vi "PXImc Custom Device.Async.vi"(10 "Parameters":variant, 11 "Process":refnum<class "Process.lvclass">) -> ()   [LabVIEW 2016, in "PXImc Custom Device Engine.lvlib"]
uses:
  PXImc Custom Device Engine.lvlib
  <vilib>/NI/NIVS Inline Async API/_VS Inline Async API/Process/Process.lvclass
  Shared/Compiled.Settings.ctl
  PXImc Router/Controls/Target Type.ctl
  PXImc Router/Controls/Router - Configuration.ctl
  PXImc Router/Controls/Router/Node Block R-W Properties.ctl
  PXImc Router/Controls/Router/Block Properties.ctl
  PXImc Router/Controls/Router/Router - PXImc Properties.ctl
  PXImc Router/Controls/Router/Router - PXImc Card Properties.ctl
  PXImc Router/Controls/Node Data.ctl
  PXImc Router/Controls/Node/Node - PXImc Parameters.ctl
  PXImc Router/Controls/Node/Node - Writer Data.ctl
  PXImc Router/Controls/Node/Node Ch Properties.ctl
  PXImc Router/Controls/Data Type.ctl
  PXImc Router/Controls/Node/Node - Readers Data.ctl
  PXImc Router/Controls/Node/Node - Reader Data.ctl
  <vilib>/NI/NIVS Inline Async API/_VS Inline Async API/Process/Process.lvclass/Process.ctl
  <vilib>/NI/NIVS Inline Async API/_Data Access Engine/Access Type Classes/Read/Read.lvclass/Read.ctl
  <vilib>/NI/NIVS Inline Async API/_Data Access Engine/Access Type Classes/Write/Write.lvclass/Write.ctl
  <vilib>/NI/NIVS Inline Async API/_Data Access Engine/Data Access Engine/Methods/Write.Data.vi
  <vilib>/NI/NIVS Inline Async API/_Data Access Engine/Data Access Engine/Methods/Read.Data.vi
  <vilib>/NI/NIVS Inline Async API/_VS Inline Async API/Process/Data Member Access/Read Data Access.vi
  <vilib>/NI/NIVS Inline Async API/_VS Inline Async API/Error Handling Process/SubVIs/Error.ConvertArray.vi
  <vilib>/NI/NIVS Inline Async API/_Data Access Engine/Access Type Classes/Write/Write.ProcessData.vi
  <vilib>/NI/NIVS Inline Async API/_Data Access Engine/Access Type Classes/Read/Read.ProcessData.vi
  <vilib>/NI/NIVS Inline Async API/_Data Access Engine/Data Access Engine/Methods/Read.Lookup.vi
  <vilib>/NI/NIVS Inline Async API/_Data Access Engine/Data Access Engine/Methods/Write.Lookup.vi
  Shared/Constants.vi
  <vilib>/NI/NIVS Inline Async API/_Data Access Engine/Data Access Engine/Data Access Engine.lvclass
  PXImc Router/PXImc Router.lvlib
  Shared/PXImc Custom Device Shared.lvlib
  <vilib>/nisyscfg/nisyscfg.lvlib
  <resource>/objmgr/nicriosae.rc
  <resource>/objmgr/nisysapi.rc
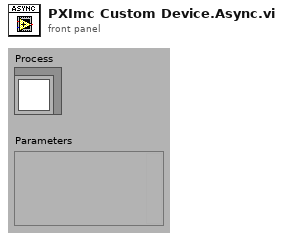
[diagram p1: front panel]
types:
  T1 = enum16{"Create File", "Log Message", "Log Error", "Log TimeStamp", "Close File"}
  T2 = typedef "PXImc Custom Device Shared.lvlib/Compiled.Settings.ctl" = cluster{"Target Type":T3, "Router Properties":T4, "Node Data":T9, "Configuration Folder Path":path}
  T3 = typedef "PXImc Router.lvlib/Target Type.ctl" = enum16{"Router", "Node"}
  T4 = typedef "PXImc Router.lvlib/Router - Configuration.ctl" = cluster{"Target Type":T3, "Master Table Ref":refnum<data-value>, "Master Table Size (Bytes)":u32, "Node Properties":T5[], "Router - PXImc Properties":T7}
  T5 = typedef "PXImc Router.lvlib/Node Block R-W Properties.ctl" = cluster{"Node ID":u32, "# Reading Blocks":u32, "Node Writing Block":T6, "Node Reading Blocks":T6[]}
  T6 = typedef "PXImc Router.lvlib/Block Properties.ctl" = cluster{"Offset":u32, "Size (Bytes)":u32}
  T7 = typedef "PXImc Router.lvlib/Router - PXImc Properties.ctl" = cluster{"PXImc Cards Properties":T8[], "Connection Timeout (s)":dbl, "Readers Buffer Size":u64}
  T8 = typedef "PXImc Router.lvlib/Router - PXImc Card Properties.ctl" = cluster{"PXImc Resource Name":string, "Reader - PXImc Session Ref":refnum<k21>, "Writer - PXImc Session Ref":refnum<k21>, "Reader Conn ID":u16, "Writer Conn ID":u16}
  T9 = typedef "PXImc Router.lvlib/Node Data.ctl" = cluster{"Node Name":string, "PXImc Parameters":T10, "Local Data":T11, "Imported Data":T14}
  T10 = typedef "PXImc Router.lvlib/Node - PXImc Parameters.ctl" = cluster{"Resource Name":string, "Connection Timeout (s)":dbl, "Readers Buffer Size":u64, "Node PXImc Reader Conn Id":u16, "Node PXImc Writer Conn Id":u16, "Writer PXImc Session":refnum<k21>, "Reader PXImc Session":refnum<k21>}
  T11 = typedef "PXImc Router.lvlib/Node - Writer Data.ctl" = cluster{"Flattened Byte Buffer Ref":string, "Noder ID":u32, "Master Table Offest":u32, "Byte Buffer Size":u32, "Node Local Channels":T12[], "Node Local Channels Table":string[][]}
  T12 = typedef "PXImc Router.lvlib/Node Ch Properties.ctl" = cluster{"Name":string, "Value":dbl, "Data Type":T13}
  T13 = typedef "PXImc Router.lvlib/Data Type.ctl" = enum16{"Boolean", "SGL", "DBL", "I8", "I16", "I32", "I64", "U8", "U16", "U32", "U64"}
  T14 = typedef "PXImc Router.lvlib/Node - Readers Data.ctl" = cluster{"Flattened Byte Buffer Ref":string, "Byte Buffer Size":u64, "Readers Data Array":T15[], "Node Imported Channels Table":string[][]}
  T15 = typedef "PXImc Router.lvlib/Node - Reader Data.ctl" = cluster{"Noder ID":u32, "Master Table Offest":u32, "Byte Buffer Size":u64, "Node Imported Channels":T12[]}
  T16 = typedef "Data Access Engine.lvlib/Data Access Engine.lvclass/Write.DVR.ctl" = refnum<data-value>
  T17 = typedef "Data Access Engine.lvlib/Data Access Engine.lvclass/Read.DVR.ctl" = refnum<data-value>
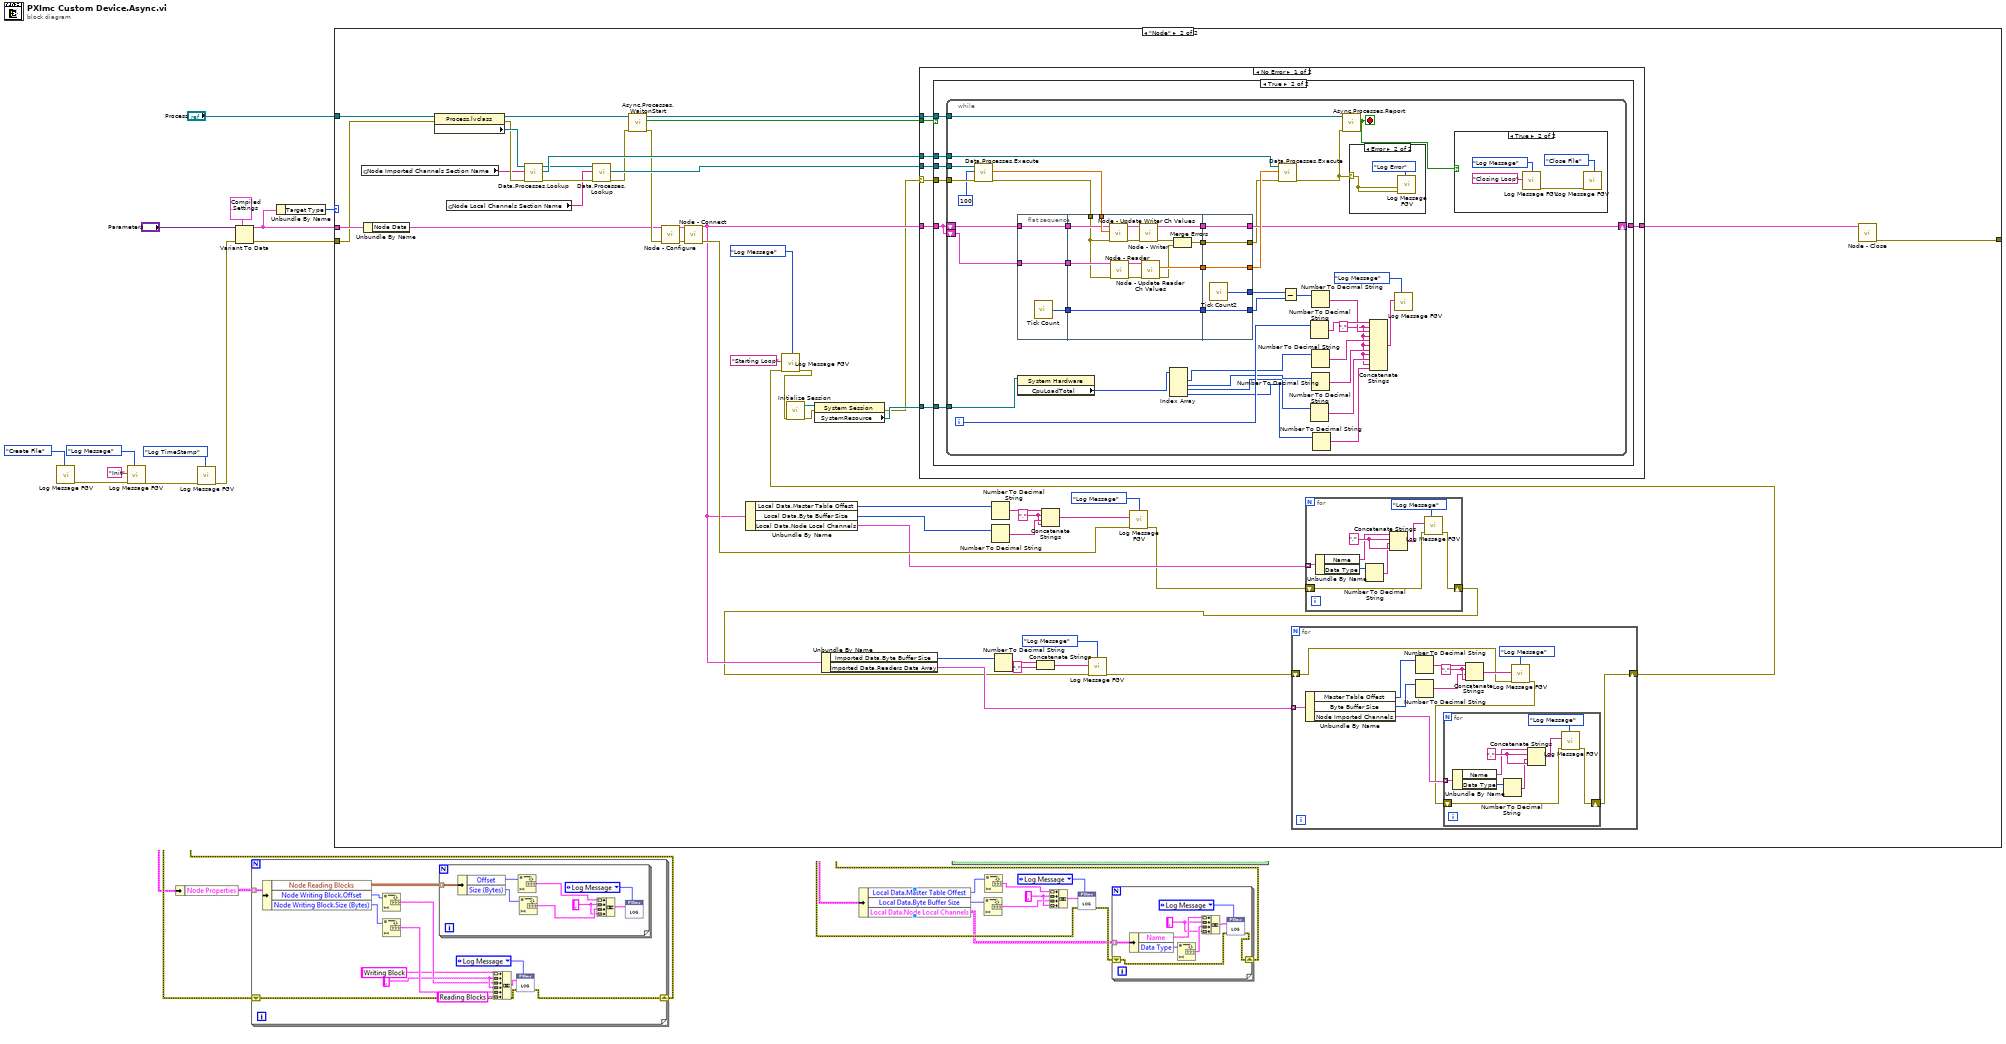
[diagram p0: block diagram]
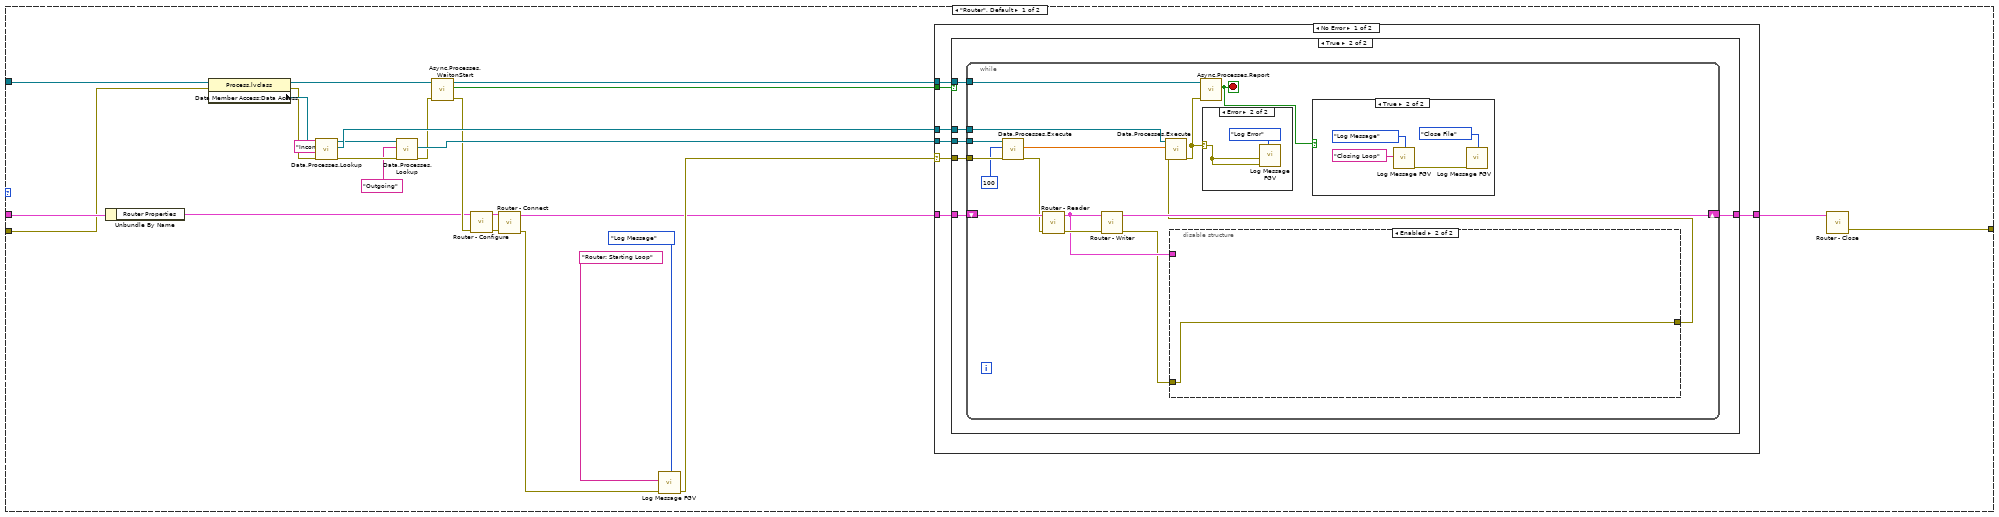
[diagram p2: hidden frame]
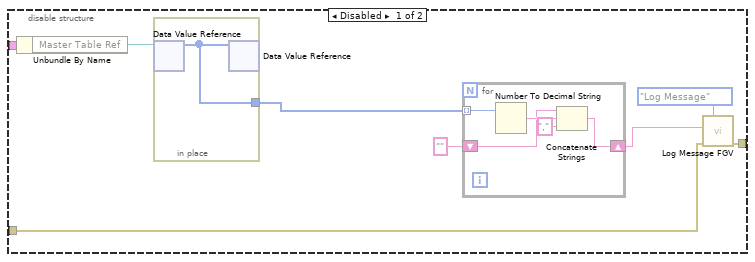
[diagram p4: hidden frame]
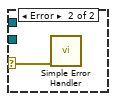
[diagram p7: hidden frame]
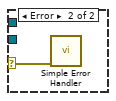
[diagram p11: hidden frame]
diagram:
  n1 = call "Log Message FGV.vi"("FGV Cmd"=T1."Create File") -> ("error out"=w7:errorcluster)  [unwired: 10 in]
  n2 = call "Log Message FGV.vi"("FGV Cmd"=T1."Log Message", "error in (no error)"=w7, "Message In"="Init") -> ("error out"=w2:errorcluster)  [unwired: 8 in]
  n3 = call "Log Message FGV.vi"("FGV Cmd"=T1."Log TimeStamp", "error in (no error)"=w2) -> ("error out"=w1:errorcluster)  [unwired: 9 in]
  n4 = Variant To Data(error in=w1, type=T2 {"Target Type"=enum."Router", "Router Properties"={"Target Type"=enum."Router", "Master Table Ref"=refnum, "Master Table Size (Bytes)"=0, "Node Properties"=[], "Router - PXImc Properties"={"PXImc Cards Properties"=[], "Connection Timeout (s)"=0.0, "Readers Buffer Size"=0}}, "Node Data"={"Node Name"="", "PXImc Parameters"={"Resource Name"="", "Connection Timeout (s)"=0.0, "Readers Buffer Size"=0, "Node PXImc Reader Conn Id"=0, "Node PXImc Writer Conn Id"=0, "Writer PXImc Session"="", "Reader PXImc Session"=""}, "Local Data"={"Flattened Byte Buffer Ref"="", "Noder ID"=0, "Master Table Offest"=0, "Byte Buffer Size"=0, "Node Local Channels"=[], "Node Local Channels Table"=[]}, "Imported Data"={"Flattened Byte Buffer Ref"="", "Byte Buffer Size"=0, "Readers Data Array"=[], "Node Imported Channels Table"=[]}}, "Configuration Folder Path"=path ""} ("Compiled.Settings"), Variant="Parameters") -> (data=w11:T2, error out=w8:errorcluster)
  n5 = Unbundle By Name(w11) -> ("Target Type"=w10:T3)
  n6 = case shown="\"Node\"" w10 {
    tunnel: "Process" -> [w35 w131]
    tunnel: w11 -> [w33 w127]
    tunnel: w8 -> [w19 w118]
    tunnel: [w22 w120] -> _
    frame "Router", Default {
      n7 = Unbundle By Name(w33) -> ("Router Properties"=w21:T4)
      n8 = property class="Process.lvclass"(reference=w35, error in=w19) -> (reference out=w34:refnum<class "Process.lvclass">, error out=w26:errorcluster, "Data Member Access:Data Access"=w27:refnum<class "Data Access Engine.lvclass">)
      n9 = call-poly <vilib>:"Data.Processes.Lookup.vi"("error in (no error)"=w26, "Name"="Incoming", "Data Access API in"=w27) -> ("error out"=w29:errorcluster, "Ref"=w36:T16, "Data Access API out"=w28:refnum<class "Data Access Engine.lvclass">)  [unwired: 5 in, 1 out]
      n10 = call-poly <vilib>:"Data.Processes.Lookup.vi"("error in (no error)"=w29, "Name"="Outgoing", "Data Access API in"=w28) -> ("error out"=w30:errorcluster, "Ref"=w37:T17)  [unwired: 5 in, 2 out]
      n11 = call <vilib>:"Async.Processes.WaitonStart.vi"("error in (no error)"=w30, "Process"=w34) -> ("error out"=w23:errorcluster, "Execute"=w39:bool, "Process out"=w38:refnum<class "Process.lvclass">)  [unwired: 7 in]
      n12 = call "Router - Configure.vi"("error in (no error)"=w23, "Router Data In"=w21) -> ("error out"=w20:errorcluster, "Router Data Out"=w31:T4)  [unwired: 8 in]
      n13 = call "Router - Connect.vi"("error in (no error)"=w20, "Router Data In"=w31) -> ("error out"=w16:errorcluster, "Router Data Out"=w14:T4)  [unwired: 8 in]
      n14 = call "Log Message FGV.vi"("FGV Cmd"=T1."Log Message", "error in (no error)"=w16, "Message In"="Router: Starting Loop") -> ("error out"=w15:errorcluster)  [unwired: 8 in]
      n15 = case shown="No Error" w15 {
        selector: w15 -> [w42 w89]
        tunnel: w39 -> [w46 _]
        tunnel: w38 -> [w45 _]
        tunnel: w36 -> [w44 _]
        tunnel: w37 -> [w43 _]
        tunnel: w14 -> [w41 _]
        tunnel: [w40 _] -> w32
        frame No Error {
          n16 = case shown="True" w46 {
            tunnel: w42 -> [_ w49]
            tunnel: w45 -> [_ w50]
            tunnel: w43 -> [_ w52]
            tunnel: w44 -> [_ w51]
            tunnel: w41 -> [_ w48]
            tunnel: [_ w47] -> w40
            frame False {
            }
            frame True {
              n17 = while {
                tunnel: w49 -> [w64]
                tunnel: w50 -> [w67]
                tunnel: w52 -> [w66]
                tunnel: w51 -> [w65]
                shift-right: [w61] -> w47
                shift-left: w48 -> [w62]
                stop <- w57 stop-if-true
                n18 = call-poly <vilib>:"Data.Processes.Execute.vi"("error in (no error)"=w64, "timeout ms"=100, "Ref"=w66) -> ("error out"=w53:errorcluster, "Values"=w63:dbl[])  [unwired: 6 in, 1 out]
                n19 = call "Router - Reader.vi"("error in (no error)"=w53, "Router Data In"=w62) -> ("error out"=w60:errorcluster, "Router Data Out"=w56:T4)  [unwired: 8 in]
                n20 = call "Router - Writer.vi"("error in (no error)"=w60, "Router Data In"=w56) -> ("error out"=w55:errorcluster, "Router Data Out"=w61:T4)  [unwired: 8 in]
                n21 = disable-structure shown="Enabled" {
                  disable-tunnel: w56 -> [w75 _]
                  disable-tunnel: w55 -> [w74 w82]
                  disable-tunnel: [w73 w82] -> w54
                  frame Disabled {
                    n22 = Unbundle By Name(w75) -> ("Master Table Ref"=w72:refnum<data-value>)
                    n23 = in-place {
                      in-place-border: [w81] -> w71
                      n24 = in-place-dvr #1(w72) -> (w81:u8[])  [unwired: 1 out]
                      n25 = in-place-dvr #1(w81) -> ()  [unwired: 2 out]
                    }
                    n26 = for {
                      shift-right: [w77] -> w68
                      shift-left: "" -> [w76]
                      tunnel: w71 -> [w80] mode=indexing
                      n27 = Number To Decimal String(number=w80) -> (decimal integer string=w79:string)  [unwired: 1 in]
                      n28 = Concatenate Strings(w76, w79, "," ("string")) -> (w77:string)
                    }
                    n29 = call "Log Message FGV.vi"("FGV Cmd"=T1."Log Message", "error in (no error)"=w74, "Message In"=w68) -> ("error out"=w73:errorcluster)  [unwired: 8 in]
                  }
                  frame Enabled {
                  }
                }
                n30 = call-poly <vilib>:"Data.Processes.Execute.vi"("error in (no error)"=w54, "Values"=w63, "Ref"=w65) -> ("error out"=w58:errorcluster)  [unwired: 8 in]
                n31 = call <vilib>:"Async.Processes.Report.vi"("Error"=w58, "Process in"=w67) -> ("Stop"=w57:bool)  [unwired: 8 in, 1 out]
                n32 = case shown="Error" w58 {
                  selector: w58 -> [_ w87]
                  frame No Error {
                  }
                  frame Error {
                    n33 = call "Log Message FGV.vi"("FGV Cmd"=T1."Log Error", "error in (no error)"=w87, "Error In"=w87) -> ()  [unwired: 8 in, 1 out]
                  }
                }
                n34 = case shown="True" w57 {
                  frame False {
                  }
                  frame True {
                    n35 = call "Log Message FGV.vi"("FGV Cmd"=T1."Log Message", "Message In"="Closing Loop") -> ("error out"=w84:errorcluster)  [unwired: 9 in]
                    n36 = call "Log Message FGV.vi"("FGV Cmd"=T1."Close File", "error in (no error)"=w84) -> ()  [unwired: 9 in, 1 out]
                  }
                }
              }
            }
          }
        }
        frame Error {
          n37 = call <vilib>:"Simple Error Handler.vi"("error in (no error)"=w89) -> ()  [unwired: 4 in, 5 out]
        }
      }
      n38 = call "Router - Close.vi"("Router Data In"=w32) -> ("error out"=w22:errorcluster)  [unwired: 10 in]
    }
    frame "Node" {
      w110 = "," ("string")
      n39 = global read "Constants.vi" "Node Imported Channels Section Name"() -> (w124:string)
      n40 = Unbundle By Name(w127) -> ("Node Data"=w115:T9)
      n41 = property class="Process.lvclass"(reference=w131, error in=w118) -> (reference out=w130:refnum<class "Process.lvclass">, error out=w128:errorcluster, "Data Member Access:Data Access"=w129:refnum<class "Data Access Engine.lvclass">)
      n42 = global read "Constants.vi" "Node Local Channels Section Name"() -> (w125:string)
      n43 = call-poly <vilib>:"Data.Processes.Lookup.vi"("error in (no error)"=w128, "Name"=w124, "Data Access API in"=w129) -> ("error out"=w134:errorcluster, "Ref"=w133:T16, "Data Access API out"=w132:refnum<class "Data Access Engine.lvclass">)  [unwired: 5 in, 1 out]
      n44 = call-poly <vilib>:"Data.Processes.Lookup.vi"("error in (no error)"=w134, "Name"=w125, "Data Access API in"=w132) -> ("error out"=w122:errorcluster, "Ref"=w135:T17)  [unwired: 5 in, 2 out]
      n45 = call <vilib>:"Async.Processes.WaitonStart.vi"("error in (no error)"=w122, "Process"=w130) -> ("error out"=w121:errorcluster, "Execute"=w137:bool, "Process out"=w136:refnum<class "Process.lvclass">)  [unwired: 7 in]
      n46 = call "Node - Configure.vi"("error in (no error)"=w121, "Node Data In"=w115) -> ("error out"=w119:errorcluster, "Node Data Out"=w123:T9)  [unwired: 8 in]
      n47 = call "Node - Connect.vi"("error in (no error)"=w119, "Node Data In"=w123) -> ("error out"=w107:errorcluster, "Node Data Out"=w104:T9)  [unwired: 8 in]
      n48 = Unbundle By Name(w104) -> ("Local Data.Master Table Offest"=w114:u32, "Local Data.Byte Buffer Size"=w113:u32, "Local Data.Node Local Channels"=w106:T12[])
      n49 = Unbundle By Name(w104) -> ("Imported Data.Byte Buffer Size"=w102:u64, "Imported Data.Readers Data Array"=w103:T15[])
      n50 = Number To Decimal String(number=w114) -> (decimal integer string=w112:string)  [unwired: 1 in]
      n51 = Number To Decimal String(number=w113) -> (decimal integer string=w111:string)  [unwired: 1 in]
      n52 = Number To Decimal String(number=w102) -> (decimal integer string=w98:string)  [unwired: 1 in]
      n53 = Concatenate Strings(w98, "," ("string")) -> (w101:string)
      n54 = Concatenate Strings(w112, w110, w111, w110) -> (w108:string)
      n55 = call "Log Message FGV.vi"("FGV Cmd"=T1."Log Message", "error in (no error)"=w107, "Message In"=w108) -> ("error out"=w105:errorcluster)  [unwired: 8 in]
      n56 = for {
        tunnel: w106 -> [w167] mode=indexing
        shift-right: [w159] -> w97
        shift-left: w105 -> [w160]
        w166 = "," ("string")
        n57 = Unbundle By Name(w167) -> ("Name"=w163:string, "Data Type"=w161:T13)
        n58 = Number To Decimal String(number=w161) -> (decimal integer string=w162:string)  [unwired: 1 in]
        n59 = Concatenate Strings(w163, w166, w162, w166) -> (w164:string)
        n60 = call "Log Message FGV.vi"("FGV Cmd"=T1."Log Message", "error in (no error)"=w160, "Message In"=w164) -> ("error out"=w159:errorcluster)  [unwired: 8 in]
      }
      n61 = call "Log Message FGV.vi"("FGV Cmd"=T1."Log Message", "error in (no error)"=w97, "Message In"=w101) -> ("error out"=w96:errorcluster)  [unwired: 8 in]
      n62 = for {
        tunnel: w103 -> [w149] mode=indexing
        shift-right: [w138] -> w95
        shift-left: w96 -> [w140]
        w145 = "," ("string")
        n63 = Unbundle By Name(w149) -> ("Master Table Offest"=w142:u32, "Byte Buffer Size"=w141:u64, "Node Imported Channels"=w148:T12[])
        n64 = Number To Decimal String(number=w142) -> (decimal integer string=w143:string)  [unwired: 1 in]
        n65 = Number To Decimal String(number=w141) -> (decimal integer string=w144:string)  [unwired: 1 in]
        n66 = Concatenate Strings(w143, w145, w144, w145) -> (w147:string)
        n67 = call "Log Message FGV.vi"("FGV Cmd"=T1."Log Message", "error in (no error)"=w140, "Message In"=w147) -> ("error out"=w139:errorcluster)  [unwired: 8 in]
        n68 = for {
          tunnel: w148 -> [w158] mode=indexing
          shift-right: [w150] -> w138
          shift-left: w139 -> [w151]
          w157 = "," ("string")
          n69 = Unbundle By Name(w158) -> ("Name"=w154:string, "Data Type"=w152:T13)
          n70 = Number To Decimal String(number=w152) -> (decimal integer string=w153:string)  [unwired: 1 in]
          n71 = Concatenate Strings(w154, w157, w153, w157) -> (w155:string)
          n72 = call "Log Message FGV.vi"("FGV Cmd"=T1."Log Message", "error in (no error)"=w151, "Message In"=w155) -> ("error out"=w150:errorcluster)  [unwired: 8 in]
        }
      }
      n73 = call "Log Message FGV.vi"("FGV Cmd"=T1."Log Message", "error in (no error)"=w95, "Message In"="Starting Loop") -> ("error out"=w94:errorcluster)  [unwired: 8 in]
      n74 = call <vilib>:"Initialize Session.vi"("error in (no error)"=w94) -> ("error out"=w90:errorcluster, "Session out"=w93:refnum<k21>)  [unwired: 9 in]
      n75 = property class="System Session"(reference=w93, error in=w90) -> (error out=w91:errorcluster, "SystemResource"=w92:refnum<k20>)  [unwired: 1 out]
      n76 = case shown="No Error" w91 {
        selector: w91 -> [w171 w251]
        tunnel: w137 -> [w175 _]
        tunnel: w136 -> [w174 _]
        tunnel: w133 -> [w173 _]
        tunnel: w135 -> [w172 _]
        tunnel: w104 -> [w170 _]
        tunnel: [w169 _] -> w126
        tunnel: w92 -> [w168 _]
        frame No Error {
          n77 = case shown="True" w175 {
            tunnel: w171 -> [_ w179]
            tunnel: w174 -> [_ w180]
            tunnel: w172 -> [_ w182]
            tunnel: w173 -> [_ w181]
            tunnel: w170 -> [_ w177]
            tunnel: [_ w178] -> w169
            tunnel: w168 -> [_ w176]
            frame False {
            }
            frame True {
              n78 = while {
                tunnel: w179 -> [w219]
                tunnel: w180 -> [w222]
                tunnel: w182 -> [w221]
                tunnel: w181 -> [w220]
                shift-right: [w211] -> w178
                shift-left: w177 -> [w213]
                shift-left: w177 -> [w212]
                tunnel: w176 -> [w188]
                i -> [w198]
                stop <- w217 stop-if-true
                w190 = "," ("string")
                n79 = call-poly <vilib>:"Data.Processes.Execute.vi"("error in (no error)"=w219, "timeout ms"=100, "Ref"=w221) -> ("error out"=w210:errorcluster, "Values"=w216:dbl[])  [unwired: 6 in, 1 out]
                n80 = flat-sequence {
                  tunnel: w212 -> [w224]
                  tunnel: w213 -> [w225]
                  tunnel: [w225] -> w209
                  tunnel: [w224] -> w208
                  tunnel: [w223] -> w202
                  tunnel: w216 -> [w239]
                  tunnel: w210 -> [w227]
                  tunnel: w209 -> [w233]
                  tunnel: w208 -> [w232]
                  tunnel: [w234] -> w207
                  tunnel: [w231] -> w206
                  tunnel: [w228] -> w205
                  tunnel: [w226] -> w203
                  tunnel: w202 -> [w226]
                  tunnel: [w242] -> w194
                  tunnel: [w243] -> w211
                  tunnel: [w244] -> w214
                  tunnel: w207 -> [w244]
                  tunnel: w206 -> [w243]
                  tunnel: w205 -> [w242]
                  tunnel: [w241] -> w204
                  tunnel: w203 -> [w240]
                  tunnel: [w240] -> w201
                  frame #0 {
                    n81 = call "Tick Count"() -> ("Tick Count(uSec)"=w223:u32)
                  }
                  frame #1 {
                    n82 = call "Node - Update Writer Ch Values.vi"("error in (no error)"=w227, "Writer Channels In"=w239, "Node Data In"=w233) -> ("error out"=w237:errorcluster, "Node Data Out"=w238:T9)  [unwired: 7 in]
                    n83 = call "Node - Reader.vi"("error in (no error)"=w227, "Node Data In"=w232) -> ("error out"=w235:errorcluster, "Node Data Out"=w236:T9)  [unwired: 8 in]
                    n84 = call "Node - Writer.vi"("error in (no error)"=w237, "Node Data In"=w238) -> ("error out"=w230:errorcluster, "Node Data Out"=w231:T9)  [unwired: 8 in]
                    n85 = call "Node - Update Reader Ch Values.vi"("error in (no error)"=w235, "Node Data In"=w236) -> ("error out"=w229:errorcluster, "Reader Ch Out"=w234:dbl[])  [unwired: 7 in, 1 out]
                    n86 = Merge Errors(w230, w229) -> (w228:errorcluster)
                  }
                  frame #2 {
                    n87 = call "Tick Count2"() -> ("Tick Count(uSec)"=w241:u32)
                  }
                }
                n88 = property class="System Hardware"(reference=w188) -> ("CpuLoadTotal"=w187:u32[])  [unwired: 1 in, 2 out]
                n89 = Index Array(array=w187) -> (element #1=w186:u32, element #2=w185:u32, element #3=w184:u32, element #4=w183:u32)  [unwired: 4 in]
                n90 = call-poly <vilib>:"Data.Processes.Execute.vi"("error in (no error)"=w194, "Values"=w214, "Ref"=w220) -> ("error out"=w215:errorcluster)  [unwired: 8 in]
                n91 = Subtract(x=w204, y=w201) -> (x-y=w200:u32)
                n92 = Number To Decimal String(number=w198) -> (decimal integer string=w197:string)  [unwired: 1 in]
                n93 = Number To Decimal String(number=w184) -> (decimal integer string=w191:string)  [unwired: 1 in]
                n94 = Number To Decimal String(number=w200) -> (decimal integer string=w196:string)  [unwired: 1 in]
                n95 = Number To Decimal String(number=w186) -> (decimal integer string=w193:string)  [unwired: 1 in]
                n96 = Number To Decimal String(number=w185) -> (decimal integer string=w192:string)  [unwired: 1 in]
                n97 = Number To Decimal String(number=w183) -> (decimal integer string=w189:string)  [unwired: 1 in]
                n98 = call <vilib>:"Async.Processes.Report.vi"("Error"=w215, "Process in"=w222) -> ("Stop"=w217:bool)  [unwired: 8 in, 1 out]
                n99 = case shown="Error" w215 {
                  selector: w215 -> [_ w245]
                  frame No Error {
                  }
                  frame Error {
                    n100 = call "Log Message FGV.vi"("FGV Cmd"=T1."Log Error", "error in (no error)"=w245, "Error In"=w245) -> ()  [unwired: 8 in, 1 out]
                  }
                }
                n101 = Concatenate Strings(w197, w190, w196, w190, w193, w190, w192, w190, w191, w190, w189) -> (w195:string)
                n102 = call "Log Message FGV.vi"("FGV Cmd"=T1."Log Message", "Message In"=w195) -> ()  [unwired: 9 in, 1 out]
                n103 = case shown="True" w217 {
                  frame False {
                  }
                  frame True {
                    n104 = call "Log Message FGV.vi"("FGV Cmd"=T1."Log Message", "Message In"="Closing Loop") -> ("error out"=w248:errorcluster)  [unwired: 9 in]
                    n105 = call "Log Message FGV.vi"("FGV Cmd"=T1."Close File", "error in (no error)"=w248) -> ()  [unwired: 9 in, 1 out]
                  }
                }
              }
            }
          }
        }
        frame Error {
          n106 = call <vilib>:"Simple Error Handler.vi"("error in (no error)"=w251) -> ()  [unwired: 4 in, 5 out]
        }
      }
      n107 = call "Node - Close.vi"("Node Data In"=w126) -> ("error out"=w120:errorcluster)  [unwired: 10 in]
    }
  }
